vi "InvalidTag_ReturnsError.vi"() -> (0 "error out":errorcluster)   [LabVIEW 2017, in "ResultTree.Tests.lvlib" / "SetDuration.lvlib"]
uses:
  SetDuration.lvlib
  ResultTree/ResultTree.lvclass
  Assertion/Assertion.lvlib
panel:
  in  "Tree":string(tree)
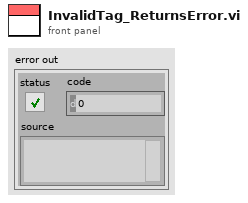
[diagram p1: front panel]
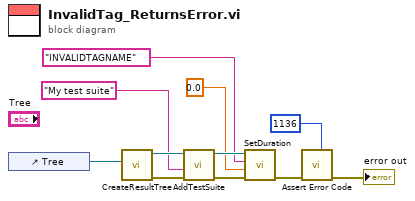
[diagram p0: block diagram]
diagram:
  n1 = control-ref of="Tree"() -> (w4:refnum<vi>)
  n2 = call "CreateResultTree.vi"("Tree Refnum"=w4) -> ("error out"=w10:errorcluster, "ResultTree out"=w9:refnum<class "ResultTree.lvclass">)  [unwired: 9 in]
  n3 = call "AddTestSuite.vi"("error in (no error)"=w10, "Name"="My test suite", "ResultTree in"=w9) -> ("error out"=w7:errorcluster, "ResultTree out"=w6:refnum<class "ResultTree.lvclass">)  [unwired: 6 in, 1 out]
  n4 = call "SetDuration.vi"("error in (no error)"=w7, "Duration [s]"=0.0, "Tag Name"="INVALIDTAGNAME", "ResultTree in"=w6) -> ("error out"=w2:errorcluster)  [unwired: 6 in, 1 out]
  n5 = call "Assert Error Code.vi"("Expected"=1136, "error in (no error)"=w2) -> ("error out"=→"error out":errorcluster)  [unwired: 9 in]
